vi "tm420_sequence_wVision.vi"() -> ()   [LabVIEW 2023, in "HamamatsuCam.lvlib" / "HamamatsuCam.lvclass"]
uses:
  HamamatsuCam/HamamatsuCam/HamamatsuCam.lvclass
panel:
  in  "Sub Region":T1={"Horizontal Offset"=0, "Vertical Offset"=0, "Horizontal Size"=1024, "Vertical Size"=1024}
  out "Display":T2(plugin-control)
  out "Timestamp":dbl
  out "DCAM Version":string
  out "Library Version":string
  out "Frames Per Second":dbl
  in  "Quit":bool
  out "Error Out":errorcluster {"code" format="%.0x"}
  # "This is just a simple example\nof how to capture and display\nlive data."
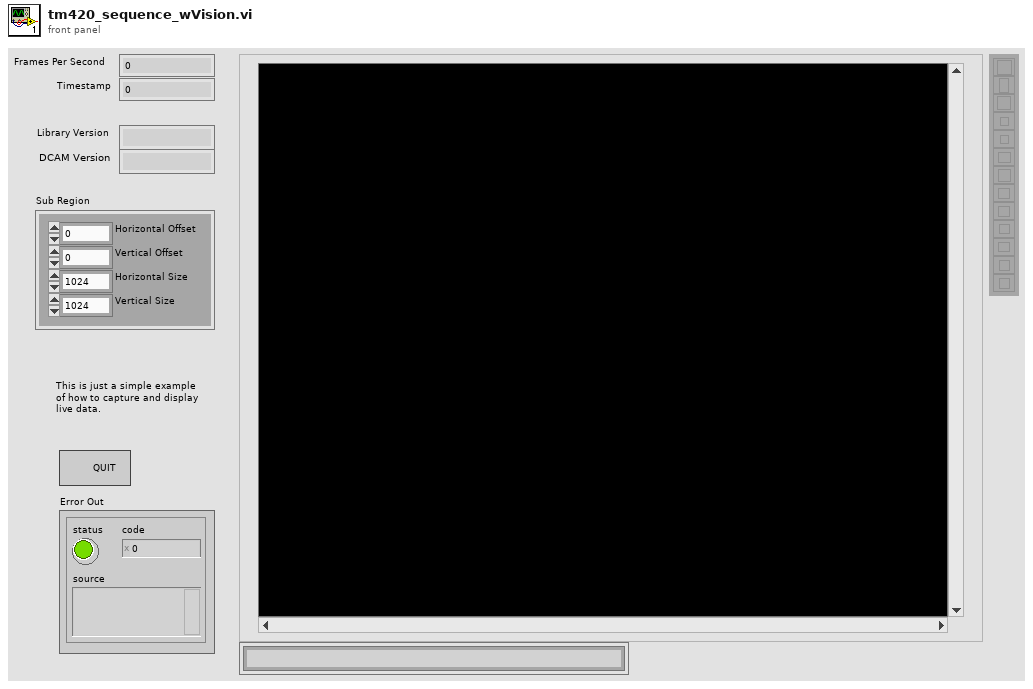
[diagram p1: front panel]
types:
  T1 = cluster{"Horizontal Offset":i32, "Vertical Offset":i32, "Horizontal Size":i32, "Vertical Size":i32}
  T2 = typedef "IMAQ Image.ctl" = refnum<image>
  T3 = cluster{"Capture Library":string, "DCAM-API":string}
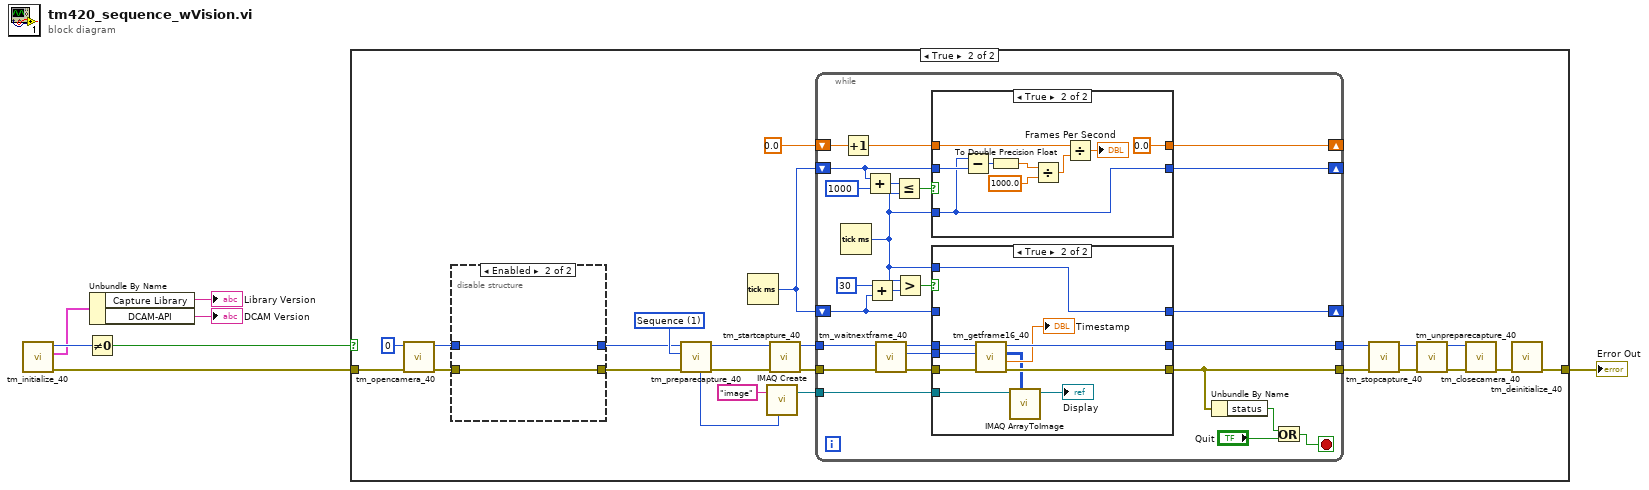
[diagram p0: block diagram]
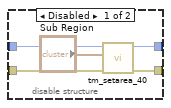
[diagram p3: hidden frame]
diagram:
  n1 = call "tm_initialize_40.vi"() -> ("error out"=w4:errorcluster, "Version Info"=w3:T3, "Number Of Cameras"=w5:u32)  [unwired: 8 in, 1 out]
  n2 = Not Equal To 0?(x=w5) -> (x != 0?=w7:bool)
  n3 = Unbundle By Name(w3) -> ("Capture Library"=→"Library Version":string, "DCAM-API"=→"DCAM Version":string)
  n4 = case shown="True" w7 {
    tunnel: w4 -> [w8 w32]
    tunnel: [w8 w29] -> w6
    frame False {
    }
    frame True {
      w20 = 1 items=["Snap", "Sequence"] ("Capture mode")
      n5 = call "tm_opencamera_40.vi"("error in (no error)"=w32, "Camera Index"=u32 0) -> ("error out"=w12:errorcluster, "Handle out"=w11:u32)  [unwired: 7 in, 1 out]
      n6 = disable-structure shown="Enabled" {
        disable-tunnel: w12 -> [w37 w38]
        disable-tunnel: w11 -> [w36 w39]
        disable-tunnel: [w35 w39] -> w10
        disable-tunnel: [w34 w38] -> w9
        frame Disabled {
          n7 = call "tm_setarea_40.vi"("error in (no error)"=w37, "Sub Region"="Sub Region", "Handle in"=w36) -> ("error out"=w34:errorcluster, "Handle out"=w35:u32)  [unwired: 7 in]
        }
        frame Enabled {
        }
      }
      n8 = call "tm_preparecapture_40.vi"("error in (no error)"=w9, "Capture mode"=w20, "Handle in"=w10) -> ("error out"=w18:errorcluster, "Handle out"=w19:u32, "Image type"=w14:u32)  [unwired: 5 in, 1 out]
      n9 = Tick Count (ms)() -> (millisecond timer value=w16:u32)
      n10 = call "IMAQ Create"("Image Name"="image", "Image Type"=w14) -> ("New Image"=w13:T2)  [unwired: 3 in, 1 out]
      n11 = call "tm_startcapture_40.vi"("error in (no error)"=w18, "Handle in"=w19) -> ("error out"=w21:errorcluster, "Handle out"=w22:u32)  [unwired: 8 in]
      n12 = while {
        tunnel: [w43] -> w25
        tunnel: [w44] -> w26
        tunnel: w22 -> [w61]
        tunnel: w21 -> [w62]
        shift-right: [w59] -> _
        shift-left: w16 -> [w56]
        shift-right: [w60] -> _
        shift-left: 0.0 -> [w53]
        shift-right: [w42] -> _
        shift-left: w16 -> [w45]
        tunnel: w13 -> [w41]
        stop <- w40 stop-if-true
        n13 = Tick Count (ms)() -> (millisecond timer value=w46:u32)
        n14 = Increment(x=w53) -> (x+1=w54:dbl)
        n15 = Add(x=w56, y=u32 1000) -> (x+y=w58:u32)
        n16 = Add(x=u32 30, y=w45) -> (x+y=w48:u32)
        n17 = call "tm_waitnextframe_40.vi"("error in (no error)"=w62, "Handle in"=w61) -> ("error out"=w51:errorcluster, "Frame Index"=w50:i32, "Handle out"=w52:u32)  [unwired: 6 in, 1 out]
        n18 = Less Or Equal?(x=w58, y=w46) -> (x <= y?=w55:bool)
        n19 = Greater?(x=w46, y=w48) -> (0:w47:bool)
        n20 = case shown="True" w55 {
          tunnel: w56 -> [w79 w82]
          tunnel: [w79 w80] -> w59
          tunnel: w54 -> [w78 w86]
          tunnel: w46 -> [_ w80]
          tunnel: [w78 0.0] -> w60
          frame False {
          }
          frame True {
            n21 = Subtract(x=w80, y=w82) -> (x-y=w81:u32)
            n22 = To Double Precision Float(number=w81) -> (double precision float=w88:dbl)
            n23 = Divide(x=w88, y=1000.0) -> (x/y=w85:dbl)
            n24 = Divide(x=w86, y=w85) -> (x/y=→"Frames Per Second":dbl)
          }
        }
        n25 = case shown="True" w47 {
          tunnel: w52 -> [w67 w77]
          tunnel: w51 -> [w66 w76]
          tunnel: w50 -> [_ w71]
          tunnel: w45 -> [w65 _]
          tunnel: w46 -> [_ w75]
          tunnel: [w67 w73] -> w43
          tunnel: [w66 w74] -> w44
          tunnel: [w65 w75] -> w42
          tunnel: w41 -> [_ w70]
          frame False {
          }
          frame True {
            n26 = call "tm_getframe16_40.vi"("error in (no error)"=w76, "Frame Index"=w71, "Handle in"=w77) -> ("error out"=w74:errorcluster, "Timestamp"=→"Timestamp":dbl, "Data"=w69:u16[][], "Handle out"=w73:u32)  [unwired: 5 in]
            n27 = call "IMAQ ArrayToImage"("Image Pixels (U16)"=w69, "Image"=w70) -> ("Image Out"=→"Display":T2)  [unwired: 8 in, 1 out]
          }
        }
        n28 = Unbundle By Name(w44) -> ("status"=w64:bool)
        n29 = Or(x=w64, y="Quit") -> (x .or. y?=w40:bool)
      }
      n30 = call "tm_stopcapture_40.vi"("error in (no error)"=w26, "Handle in"=w25) -> ("error out"=w23:errorcluster, "Handle out"=w24:u32)  [unwired: 8 in]
      n31 = call "tm_unpreparecapture_40.vi"("error in (no error)"=w23, "Handle in"=w24) -> ("error out"=w28:errorcluster, "Handle out"=w27:u32)  [unwired: 8 in]
      n32 = call "tm_closecamera_40.vi"("error in (no error)"=w28, "Handle in"=w27) -> ("error out"=w30:errorcluster)  [unwired: 9 in]
      n33 = call "tm_deinitialize_40.vi"("error in (no error)"=w30) -> ("error out"=w29:errorcluster)  [unwired: 10 in]
    }
  }
  "Error Out" <- w6
